vi "Shooter Controller.vi"(8 "error in":errorcluster) -> ()   [LabVIEW 2016]
doc: "This VI executes continuously carrying out the current operation and responding to updates or new operations. It will often contain the timing or control code that is difficult to place directly in TeleOp. This VI generally opens all sensors and motors and isolates the rest of the robot code from knowing how the operations are carried out."
uses:
  Shooter Setpoints.ctl
  Shooter Operations.ctl
  <vilib>/Rock Robotics/WPI/SafetyOutput/WPI_SafetyOutputConfigMenu.ctl
  <vilib>/Rock Robotics/SystemInterfaces/DIO/FPGA_DIOPWMChannel.ctl
  <vilib>/Rock Robotics/WPI/MotorControl/WPI_MotorControlOpen Talon.vi
  <vilib>/Rock Robotics/Network Tables/NT Write Boolean.vi
panel:
  out "Current\nCmd":string
  # "Tip: It may be helpful to observe inputs and sensor values.\nYou may also want to display tuning or debugging controls."
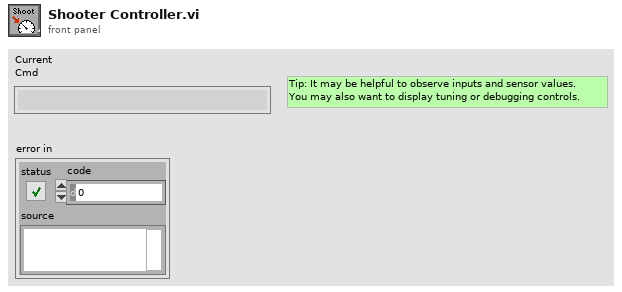
[diagram p1: front panel]
types:
  T1 = typedef "FPGA_DIOPWMChannel.ctl" = enum8{"PWM 0", "PWM 1", "PWM 2", "PWM 3", "PWM 4", "PWM 5", "PWM 6", "PWM 7", "PWM 8", "PWM 9", "PWM MXP 0", "PWM MXP 1", "PWM MXP 2", "PWM MXP 3", "PWM MXP 4", "PWM MXP 5", "PWM MXP 6", "PWM MXP 7", "PWM MXP 8", "PWM MXP 9", "Invalid"}
  T2 = typedef "WPI_SafetyOutputConfigMenu.ctl" = enum16{"Enable", "Disable"}
  T3 = typedef "Shooter Setpoints.ctl" = cluster{"Operation":T4, "Setpoint":dbl, "Duration":dbl}
  T4 = typedef "Shooter Operations.ctl" = enum16{"Reserve", "Read Current", "Immediate", "Shooter Toggle"}
  T5 = typedef "WPI_MotorControlDeviceRef.ctl" = cluster{"DeviceStatus":errorcluster, "Type":T6, "PWM":cluster{"PWM Channel":T1, "DeadBand":T7}, "CAN":cluster{"Device Number":u8, "SetOutput VI Ref":variant, "GetOutput VI Ref":variant, "Enable VI Ref":variant, "Disable VI Ref":variant, "Data":variant}, "Invert":bool}
  T6 = typedef "WPI_MotorControlType.ctl" = enum16{"PWM", "CAN"}
  T7 = typedef "WPI_PWMDeadband.ctl" = cluster{"Name":string, "maxPositivePwm":i32, "minPositivePwm":i32, "centerPwm":i32, "maxNegativePwm":i32, "minNegativePwm":i32, "angularRange":u16}
  T8 = typedef "Command Status Info.ctl" = cluster{"Name":string, "Status":T9, "notifier out":T10}
  T9 = typedef "Completion Status.ctl" = enum16{"Successful", "Aborted", "Incomplete"}
  T10 = typedef "Completion Notifier.ctl" = refnum<notifier>
  T11 = cluster{"Default Command":T3, "Command Timing":cluster{"Start Time (ms)":u32, "Iterations":i32}, "Command Arguments":cluster{"Command Info":T8, "Description":string, "Default Command":T3, "notifier out":refnum<notifier>, "Subsystem Name":string}}
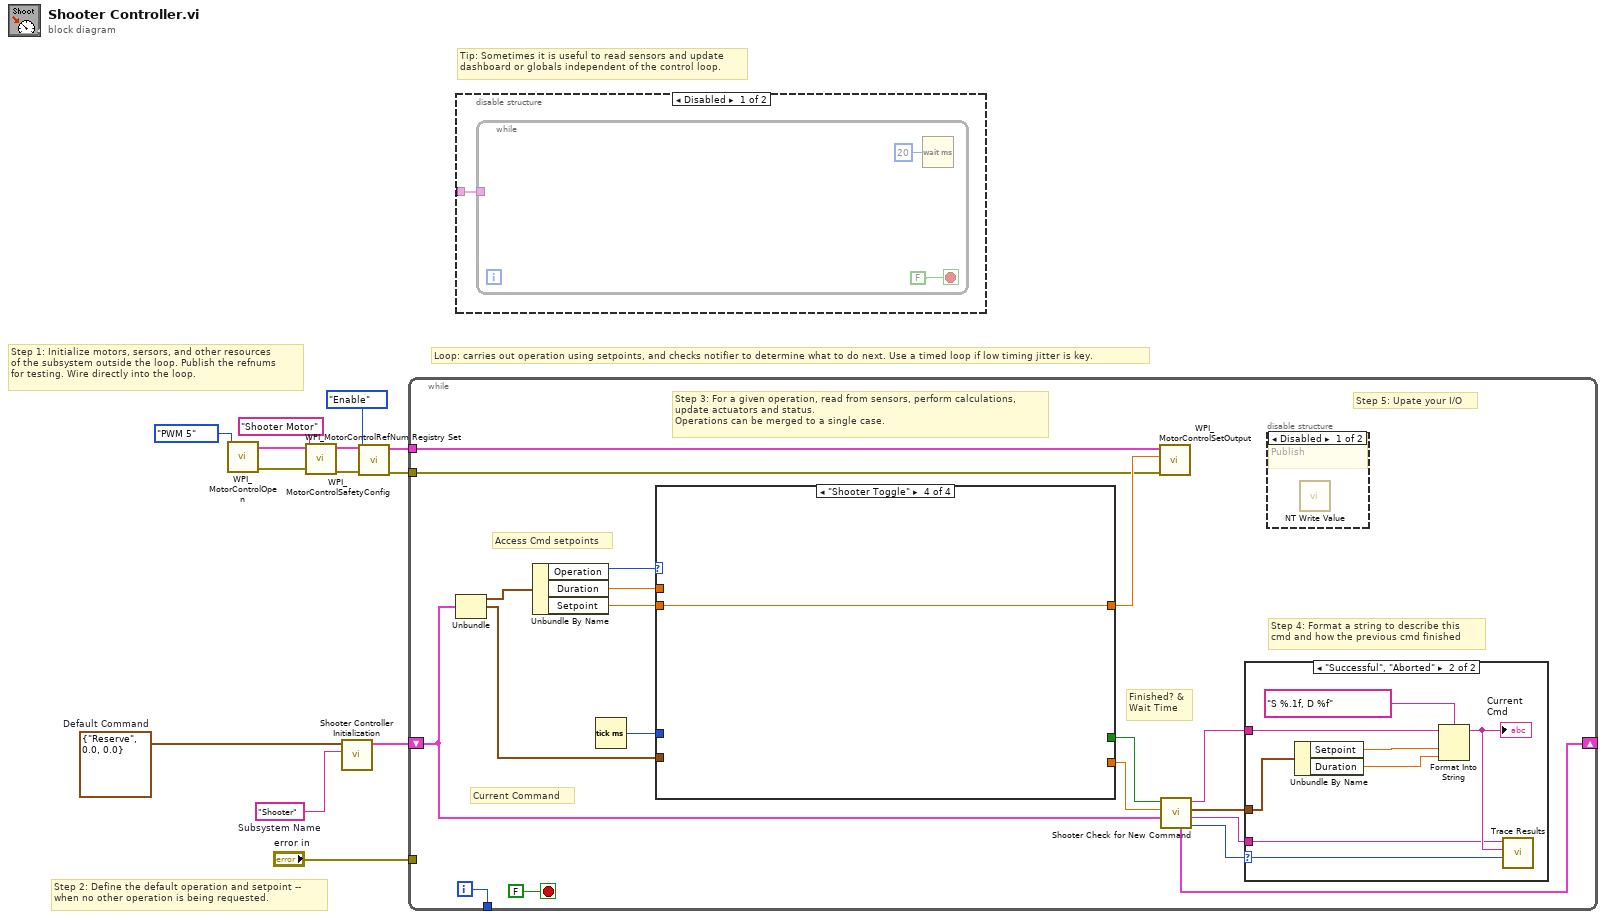
[diagram p0: block diagram]
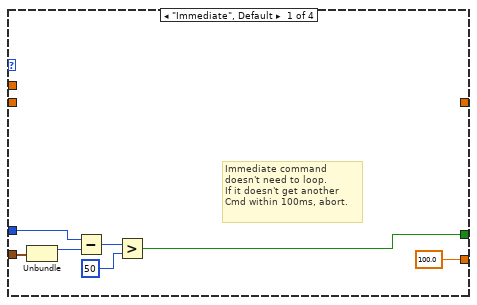
[diagram p5: hidden frame]
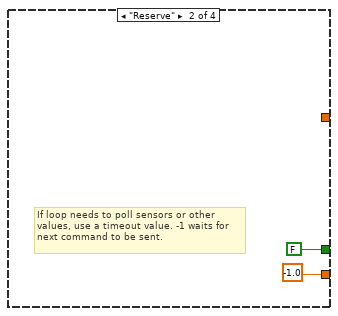
[diagram p6: hidden frame]
diagram:
  w10 = T3 {"Operation"=enum."Reserve", "Setpoint"=0.0, "Duration"=0.0}  # Default Command
  w11 = "Shooter"  # Subsystem Name
  # "Tip: Sometimes it is useful to read sensors and update\ndashboard or globals independent of the control loop."
  # "Step 2: Define the default operation and setpoint --\nwhen no other operation is being requested."
  # "Step 1: Initialize motors, sersors, and other resources\nof the subsystem outside the loop. Publish the refnums\nfor testing. Wire directly into the loop."
  # "Loop: carries out operation using setpoints, and checks notifier to determine what to do next. Use a timed loop if low timing jitter is key."
  n1 = call-poly <vilib>:"WPI_MotorControlOpen.vi"("PWM Channel"=FPGA_DIOPWMChannel."PWM 5") -> ("error out"=w7:errorcluster, "MotorControlDeviceRef"=w9:T5)  [unwired: 9 in]
  n2 = call <vilib>:"WPI_MotorControlRefNum Registry Set.vi"("error in (no error)"=w7, "refnum name"="Shooter Motor", "MotorControlDevRef"=w9) -> ("error out"=w6:errorcluster, "MotorControlDevRef"=w5:T5)  [unwired: 7 in]
  n3 = call "Shooter Controller Initialization.vi"("Subsystem Name"=w11, "Default Command"=w10) -> ("Command Info"=w12:T11)  [unwired: 9 in]
  n4 = call <vilib>:"WPI_MotorControlSafetyConfig.vi"("error in (no error)"=w6, "mode"=WPI_SafetyOutputConfigMenu."Enable", "MotorControlDevRef"=w5) -> ("error out"=w3:errorcluster, "MotorControlDevRef"=w4:T5)  [unwired: 7 in]
  n5 = while {
    shift-right: [w23] -> _
    shift-left: w12 -> [w24]
    tunnel: [w31] -> _
    tunnel: "error in" -> [_]
    tunnel: w4 -> [w16]
    tunnel: w3 -> [w14]
    i -> [w31]
    stop <- FALSE stop-if-true
    # "Step 5: Upate your I/O"
    # "Step 4: Format a string to describe this\ncmd and how the previous cmd finished"
    # "Current Command"
    # "Access Cmd setpoints"
    # "Finished? &\nWait Time"
    # "Step 3: For a given operation, read from sensors, perform calculations,\nupdate actuators and status.\nOperations can be merged to a single case."
    n6 = Unbundle(w24) -> ("Default Command"=w30:T3, "Command Timing"=w26:cluster{"Start Time (ms)":u32, "Iterations":i32})  [unwired: 1 out]
    n7 = Unbundle By Name(w30) -> ("Operation"=w29:T4, "Duration"=w28:dbl, "Setpoint"=w25:dbl)
    n8 = Tick Count (ms)() -> (millisecond timer value=w27:u32)
    n9 = case shown="\"Shooter Toggle\"" w29 {
      tunnel: [100.0 -1.0 _ _] -> w21
      tunnel: [w41 FALSE ("ignore previous (F)") _ _] -> w22
      tunnel: w26 -> [w43 _ _ _]
      tunnel: w28 -> [_ _ _ _]
      tunnel: w27 -> [w42 _ _ _]
      tunnel: w25 -> [_ _ _ w50]
      tunnel: [_ _ _ w50] -> w15
      frame "Immediate", Default {
        # "Immediate command\ndoesn't need to loop.\nIf it doesn't get another\nCmd within 100ms, abort."
        n10 = Unbundle(w43) -> ("Start Time (ms)"=w46:u32)  [unwired: 1 out]
        n11 = Subtract(x=w42, y=w46) -> (x-y=w45:u32)
        n12 = Greater?(x=w45, y=u8 50 ("Left Motor")) -> (0:w41:bool)
      }
      frame "Reserve" {
        # "If loop needs to poll sensors or other\nvalues, use a timeout value. -1 waits for\nnext command to be sent."
      }
      frame "Read Current" {
      }
      frame "Shooter Toggle" {
      }
    }
    n13 = call <vilib>:"WPI_MotorControlSetOutput.vi"("error in (no error)"=w14, "Output"=w15, "MotorControlDevRef"=w16) -> ()  [unwired: 6 in, 3 out]
    n14 = call "Shooter Check for New Command.vi"("Current Command"=w24, "Wait time (ms)"=w21, "Finished?"=w22) -> ("Completion"=w17:T9, "Subsystem Name"=w18:string, "Current Command"=w19:T3, "Initial Trace String"=w20:string, "NextCommand"=w23:T11)  [unwired: 4 in]
    n15 = case shown="\"Successful\", \"Aborted\"" w17 {
      selector: w17 -> [_ w40]
      tunnel: w20 -> [_ w36]
      tunnel: w19 -> [_ w37]
      tunnel: w18 -> [_ w33]
      frame "Incomplete", Default {
        # "Continuing current command"
      }
      frame "Successful", "Aborted" {
        # "Report and setup for next command"
        n16 = Unbundle By Name(w37) -> ("Setpoint"=w39:dbl, "Duration"=w34:dbl)
        n17 = Format Into String(format string="S %.1f, D %f", initial string=w36, w39, w34) -> (resulting string=w35:string)  [unwired: 1 in, 1 out]
        "Current\nCmd" <- w35
        n18 = call <vilib>:"Trace Results.vi"("Status of previous command"=w40, "Description"=w35, "Subsystem"=w33) -> ()  [unwired: 9 in]
      }
    }
    n19 = disable-structure shown="Disabled" {
      frame Disabled {
        # "Publish"
        n20 = call-poly <vilib>:"NT Write Value.vi"() -> ()  [unwired: 11 in, 1 out]
      }
      frame Enabled {
      }
    }
  }
  n21 = disable-structure shown="Disabled" {
    disable-tunnel: _ -> [w51 _]
    frame Disabled {
      n22 = while {
        tunnel: w51 -> [_]
        stop <- FALSE stop-if-true
        n23 = Wait (ms)(milliseconds to wait=u32 20) -> ()  [unwired: 1 out]
      }
    }
    frame Enabled {
    }
  }
